vi "hse-configuration_ReadIntegerKey.vi"(8 "error in (no error)":errorcluster, 9 "Key":string, 10 "Section":string, 11 "hse-config-ini in":refnum<class "hse-config-ini.lvclass">) -> (0 "error out":errorcluster, 2 "Value":i32, 3 "hse-config-ini out":refnum<class "hse-config-ini.lvclass">)   [LabVIEW 2014, in "hse-config-ini.lvclass"]
doc: "Reads the numeric configuration value (I32) identified by <b>section</b> and <b>key</b> from the configuration object"
uses:
  hse-config-ini.lvclass
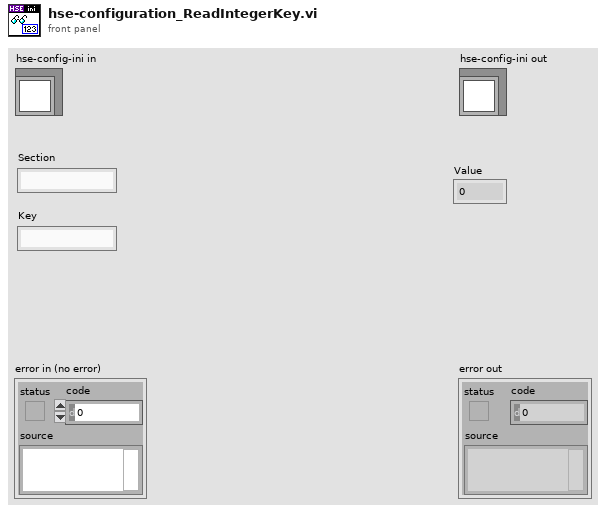
[diagram p1: front panel]
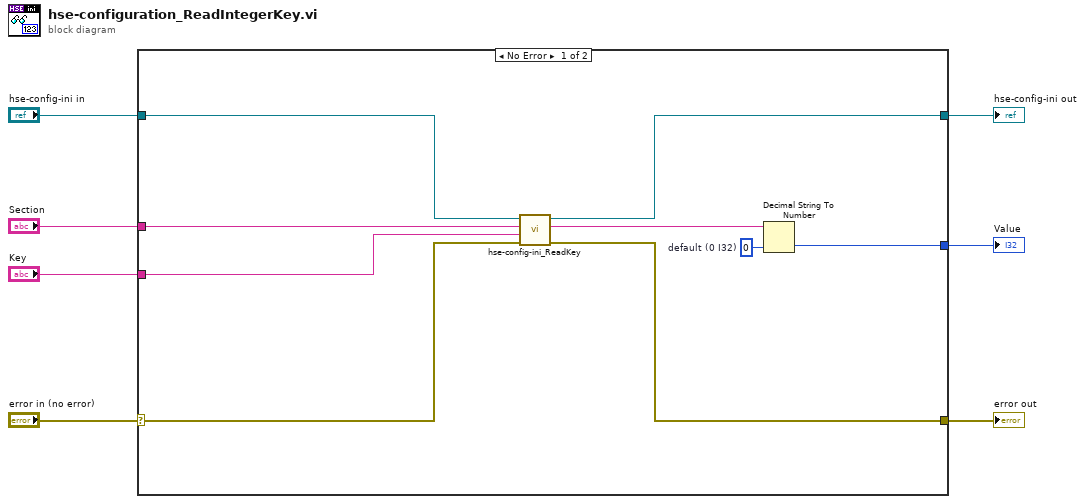
[diagram p0: block diagram]
diagram:
  n1 = case shown="No Error" "error in (no error)" {
    selector: "error in (no error)" -> [w12 w18]
    tunnel: [w11 w18] -> w7
    tunnel: "hse-config-ini in" -> [w16 w17]
    tunnel: [w15 w17] -> w4
    tunnel: "Section" -> [w14 _]
    tunnel: "Key" -> [w13 _]
    tunnel: [w9 _] -> w6
    frame No Error {
      w8 = 0  # default (0 I32)
      n2 = call "hse-config-ini_ReadKey.vi"("error in (no error)"=w12, "Key"=w13, "Section"=w14, "hse-config-ini in"=w16) -> ("error out"=w11:errorcluster, "String"=w10:string, "hse-config-ini out"=w15:refnum<class "hse-config-ini.lvclass">)  [unwired: 5 in]
      n3 = Decimal String To Number(string=w10, default (0L)=w8) -> (number=w9:i32)  [unwired: 1 in, 1 out]
    }
    frame Error {
    }
  }
  "error out" <- w7
  "hse-config-ini out" <- w4
  "Value" <- w6
